vi "FPGA_Host_USB7855R.vi"() -> (8 "FilePath":path=path "D:/temp/test.tdms")   [LabVIEW 2023]
uses:
  <vilib>/rvi/interface/nirviReadWriteControl/nirviReadWriteControl.xnode
  <vilib>/rvi/interface/nirviMethod/nirviMethod.xnode
  User_Vi/Settings.vi
  <vilib>/rvi/interface/nirviOpenFPGA/nirviOpenFPGA.xnode
  <vilib>/rvi/errors/niLvFpgaMergeErrorWithErrorCode.vi
  <vilib>/rvi/errors/niLvFpgaAdjustHostInterfaceError.vi
  AllFiles_WEC-SPM-master/AllFiles_WEC-SPM-master/Sub_Vi/FPGA/FPGA_Target_USB_7855R.vi
  AllFiles_WEC-SPM-master/AllFiles_WEC-SPM-master/FPGA Bitfiles/wecspmusb7855r_FPGATargetUSB785_FPGATargetUSB785_scBLrgoL084.lvbitx
  <vilib>/FPGAPlugInAG/Dynamic/niLvFpga_Run_Dynamic.vi
  <vilib>/rvi/interface/Simulation/niFpgaSimulationCallBeginRW.vi
  <vilib>/FPGAPlugInAG/Dynamic/niLvFpga_WriteFifo_Dynamic.vi
  <vilib>/FPGAPlugInAG/Dynamic/niLvFpga_ReadFifo_Dynamic.vi
  <vilib>/FPGAPlugInAG/Dynamic/niLvFpga_StartFifo_Dynamic.vi
  <vilib>/FPGAPlugInAG/Dynamic/niLvFpga_StopFifo_Dynamic.vi
  TypeDefs/WayPointCluster.ctl
  TypeDefs/Settings.ctl
  TypeDefs/ChangeOnFly.ctl
  TypeDefs/Display.ctl
panel:
  in  "FPGA VI Reference Out":refnum<k20>
  out "error out 4":errorcluster
  out "error out 3":errorcluster
  out "Stop Hold Position":bool
  out "Applied Z":i16
  out "DIO0":bool
  out "error out 2":errorcluster
  out "error out":errorcluster
  out "ChangeonFlyUpdate":T1
  in  "Display Cluster":T2
  in  "ChangeonFly":T3
  in  "SettingsCluster":T4={"Sample Rate (us)"=1, "Samples Per Data Point (int, power of 2)"=1000, "DistanceToBulk (um)"=-1.0, "HoldTimeScaler"=1, "SaveData"=TRUE, "DistanceToBulk (um) 2"=-1.0, "DistanceToBulk (um) 3"=-1.0}
  in  "WayPointCluster":T5
  out "tdms file out":refnum<k34>
  out "ElementsToRead":u32=800
  in  "stop":bool
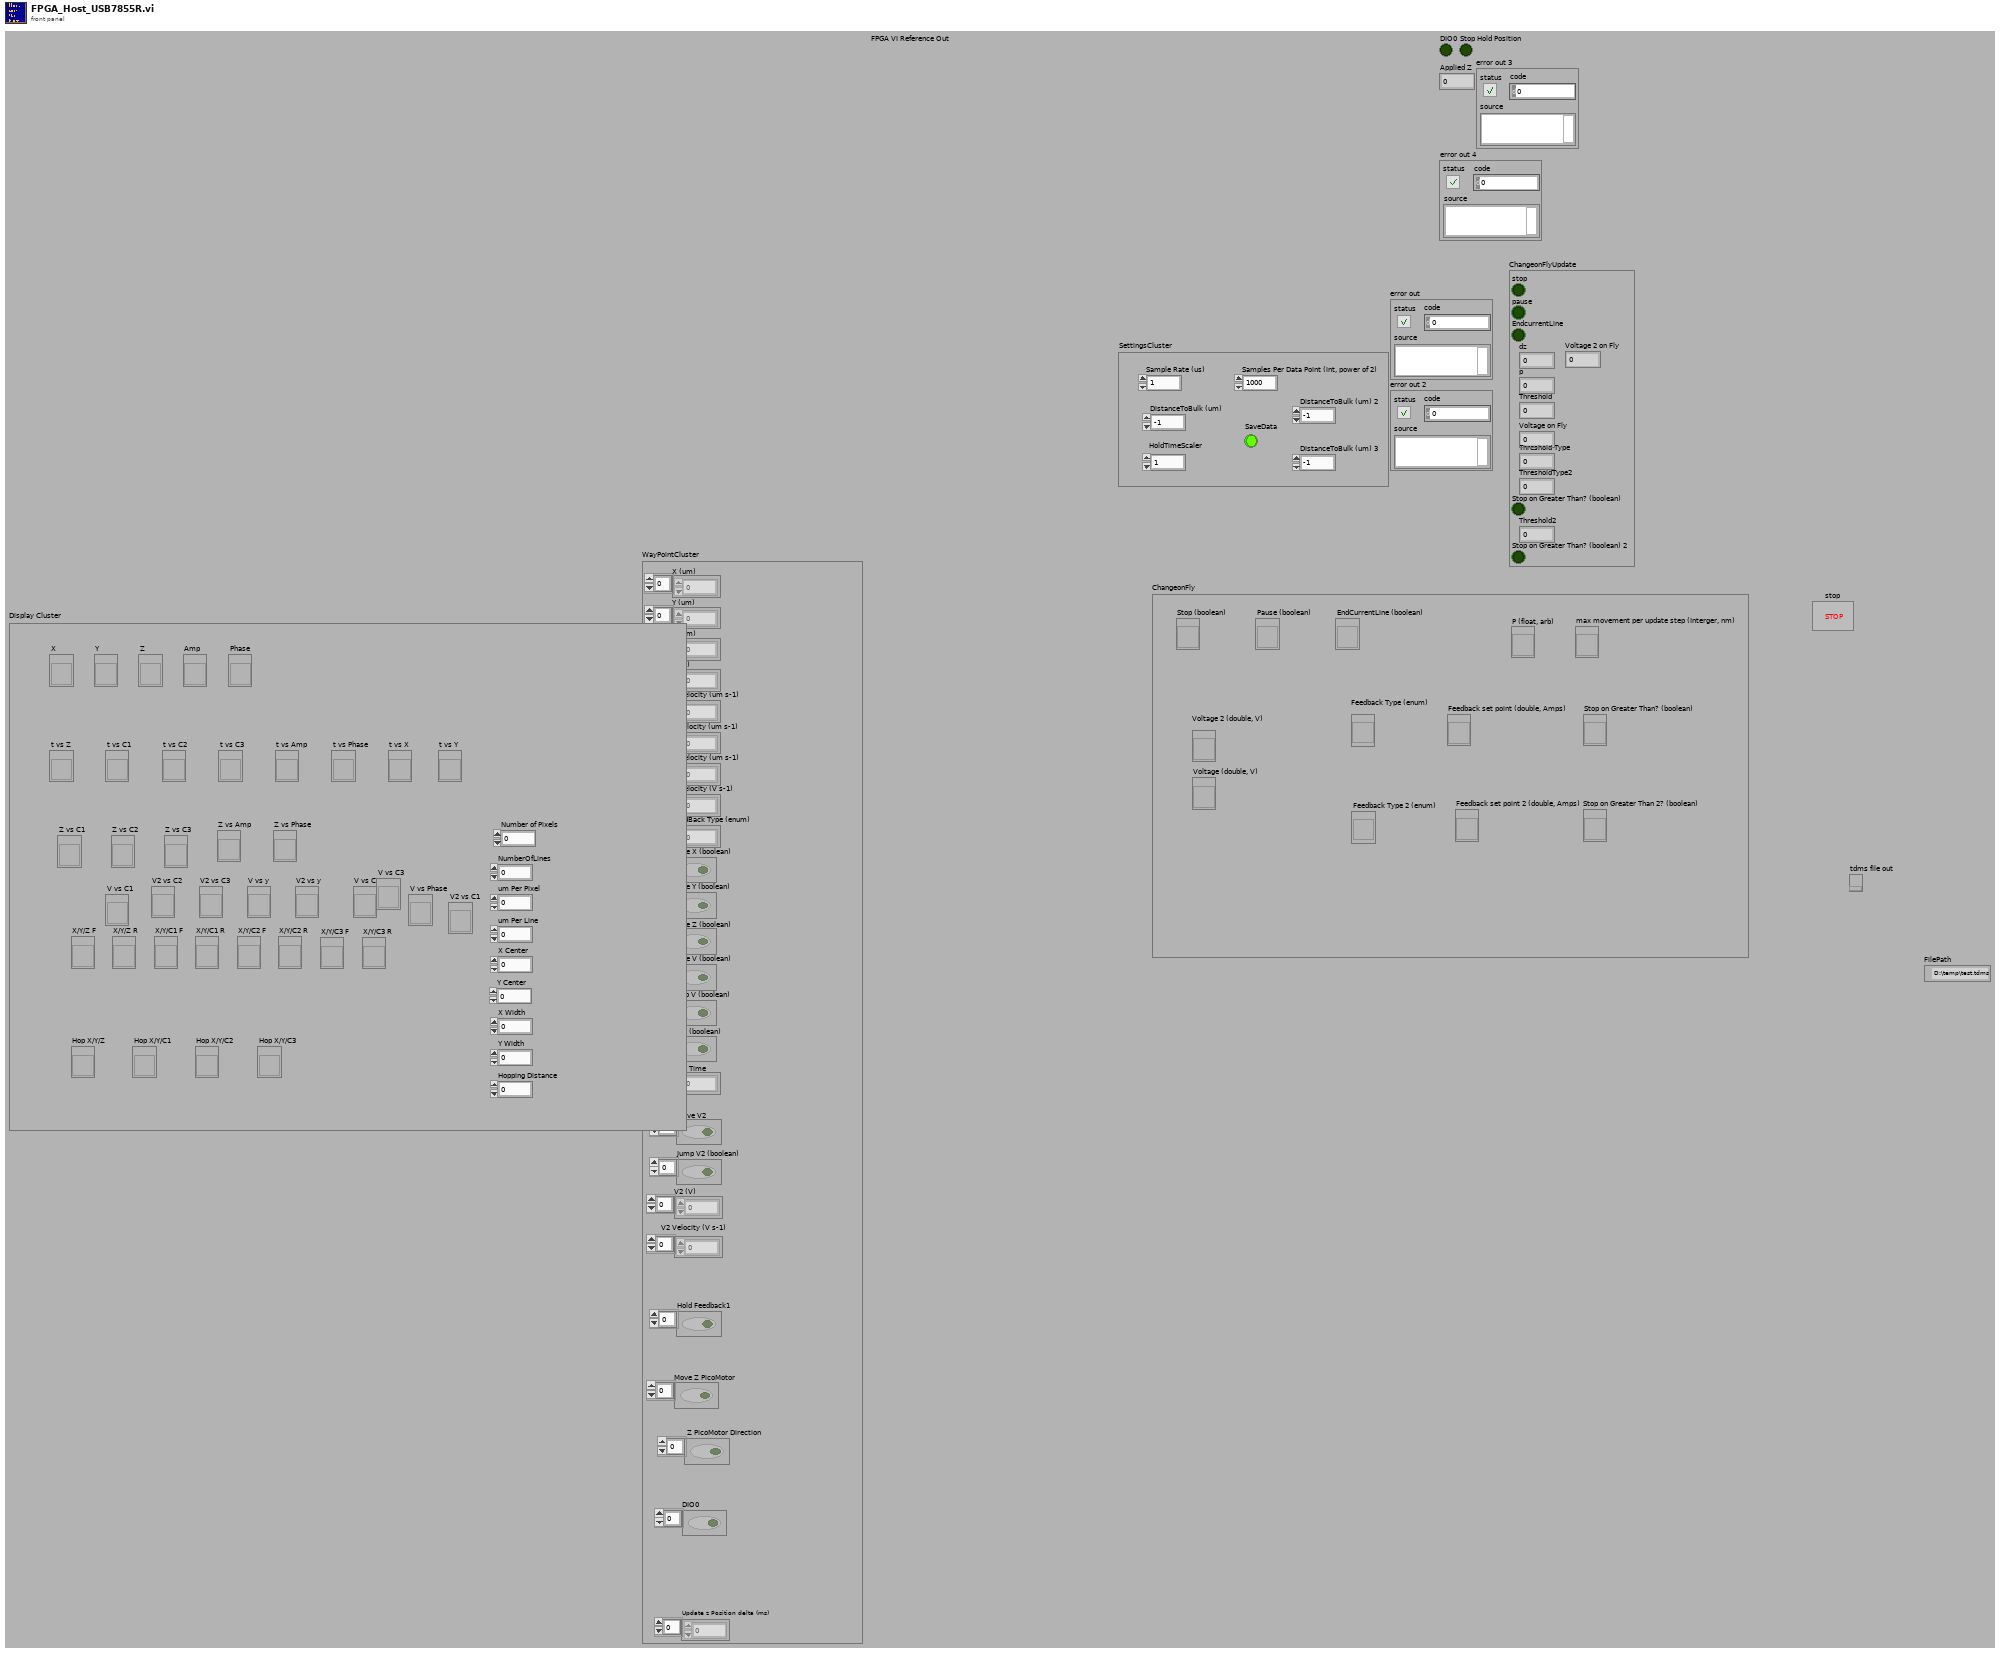
[diagram p1: front panel]
types:
  T1 = cluster{"stop":bool, "pause":bool, "EndcurrentLine":bool, "dz":i32, "p":fxp<+/-,32,1>, "Threshold":i32, "Voltage on Fly":i16, "Threshold Type":u8, "ThresholdType2":u8, "Stop on Greater Than? (boolean)":bool, "Threshold2":i32, "Stop on Greater Than? (boolean) 2":bool, "Voltage 2 on Fly":i16}
  T2 = typedef "Display.ctl" = cluster{"X":refnum<vi>, "Y":refnum<vi>, "Z":refnum<vi>, "Amp":refnum<vi>, "Phase":refnum<vi>, "t vs Z":refnum<vi>, "t vs C1":refnum<vi>, "t vs C2":refnum<vi>, "t vs C3":refnum<vi>, "t vs Amp":refnum<vi>, "t vs Phase":refnum<vi>, "t vs X":refnum<vi>, "t vs Y":refnum<vi>, "Z vs C1":refnum<vi>, "Z vs C2":refnum<vi>, "Z vs C3":refnum<vi>, "V vs C1":refnum<vi>, "V vs C2":refnum<vi>, "V vs C3":refnum<vi>, "X/Y/Z F":refnum<vi>, "X/Y/Z R":refnum<vi>, "X/Y/C1 F":refnum<vi>, "X/Y/C1 R":refnum<vi>, "X/Y/C2 F":refnum<vi>, "X/Y/C2 R":refnum<vi>, "X/Y/C3 F":refnum<vi>, "X/Y/C3 R":refnum<vi>, "NumberOfLines":u16, "um Per Pixel":dbl, "um Per Line":dbl, "X Center":dbl, "Hop X/Y/Z":refnum<vi>, "Hop X/Y/C1":refnum<vi>, "Hop X/Y/C2":refnum<vi>, "Hop X/Y/C3":refnum<vi>, "X Width":dbl, "Y Width":dbl, "Hopping Distance":dbl, "V2 vs C1":refnum<vi>, "V vs Phase":refnum<vi>, "Y Center":dbl, "Number of Pixels":dbl, "V2 vs C2":refnum<vi>, "V2 vs C3":refnum<vi>, "V vs y":refnum<vi>, "V2 vs y":refnum<vi>, "Z vs Amp":refnum<vi>, "Z vs Phase":refnum<vi>}
  T3 = typedef "ChangeOnFly.ctl" = cluster{"Stop (boolean)":refnum<vi>, "Pause (boolean)":refnum<vi>, "EndCurrentLine (boolean)":refnum<vi>, "max movement per update step (Interger, nm)":refnum<vi>, "P (float, arb)":refnum<vi>, "Feedback set point (double, Amps)":refnum<vi>, "Voltage (double, V)":refnum<vi>, "Feedback set point 2 (double, Amps)":refnum<vi>, "Stop on Greater Than 2? (boolean)":refnum<vi>, "Stop on Greater Than? (boolean)":refnum<vi>, "Voltage 2 (double, V)":refnum<vi>, "Feedback Type (enum)":refnum<vi>, "Feedback Type 2 (enum)":refnum<vi>}
  T4 = typedef "Settings.ctl" = cluster{"Sample Rate (us)":u32, "Samples Per Data Point (int, power of 2)":i16, "DistanceToBulk (um)":dbl, "HoldTimeScaler":u64, "SaveData":bool, "DistanceToBulk (um) 2":dbl, "DistanceToBulk (um) 3":dbl}
  T5 = typedef "WayPointCluster.ctl" = cluster{"X (um)":dbl[], "Y (um)":dbl[], "Z (um)":dbl[], "V (V)":dbl[], "X Velocity (um s-1)":dbl[], "Y Velocity (um s-1)":dbl[], "Z Velocity (um s-1)":dbl[], "V Velocity (V s-1)":dbl[], "FeedBack Type (enum)":u16[], "Move X (boolean)":bool[], "Move Y (boolean)":bool[], "Move Z (boolean)":bool[], "Move V (boolean)":bool[], "Jump V (boolean)":bool[], "Hold (boolean)":bool[], "Hold Time":u32[], "V2 (V)":dbl[], "Move V2":bool[], "V2 Velocity (V s-1)":dbl[], "Jump V2 (boolean)":bool[], "Update z Position delta (ms)":i16[], "Hold Feedback1":bool[], "Move Z PicoMotor":bool[], " Z PicoMotor Direction":bool[], "DIO0":bool[]}
  T6 = typedef "nirio_resource_hc.ctl" = tag
  T7 = typedef "VelScallerCluster.ctl" = cluster{"X_VelScaller":i32, "Y_VelScaller":i32, "Z_VelScaller":i32, "V s-1_VelScaller":i32, "V2 s-1_VelScaller":i32}
  T8 = enum16{"open", "open or create", "create or replace", "create", "open (read-only)"}
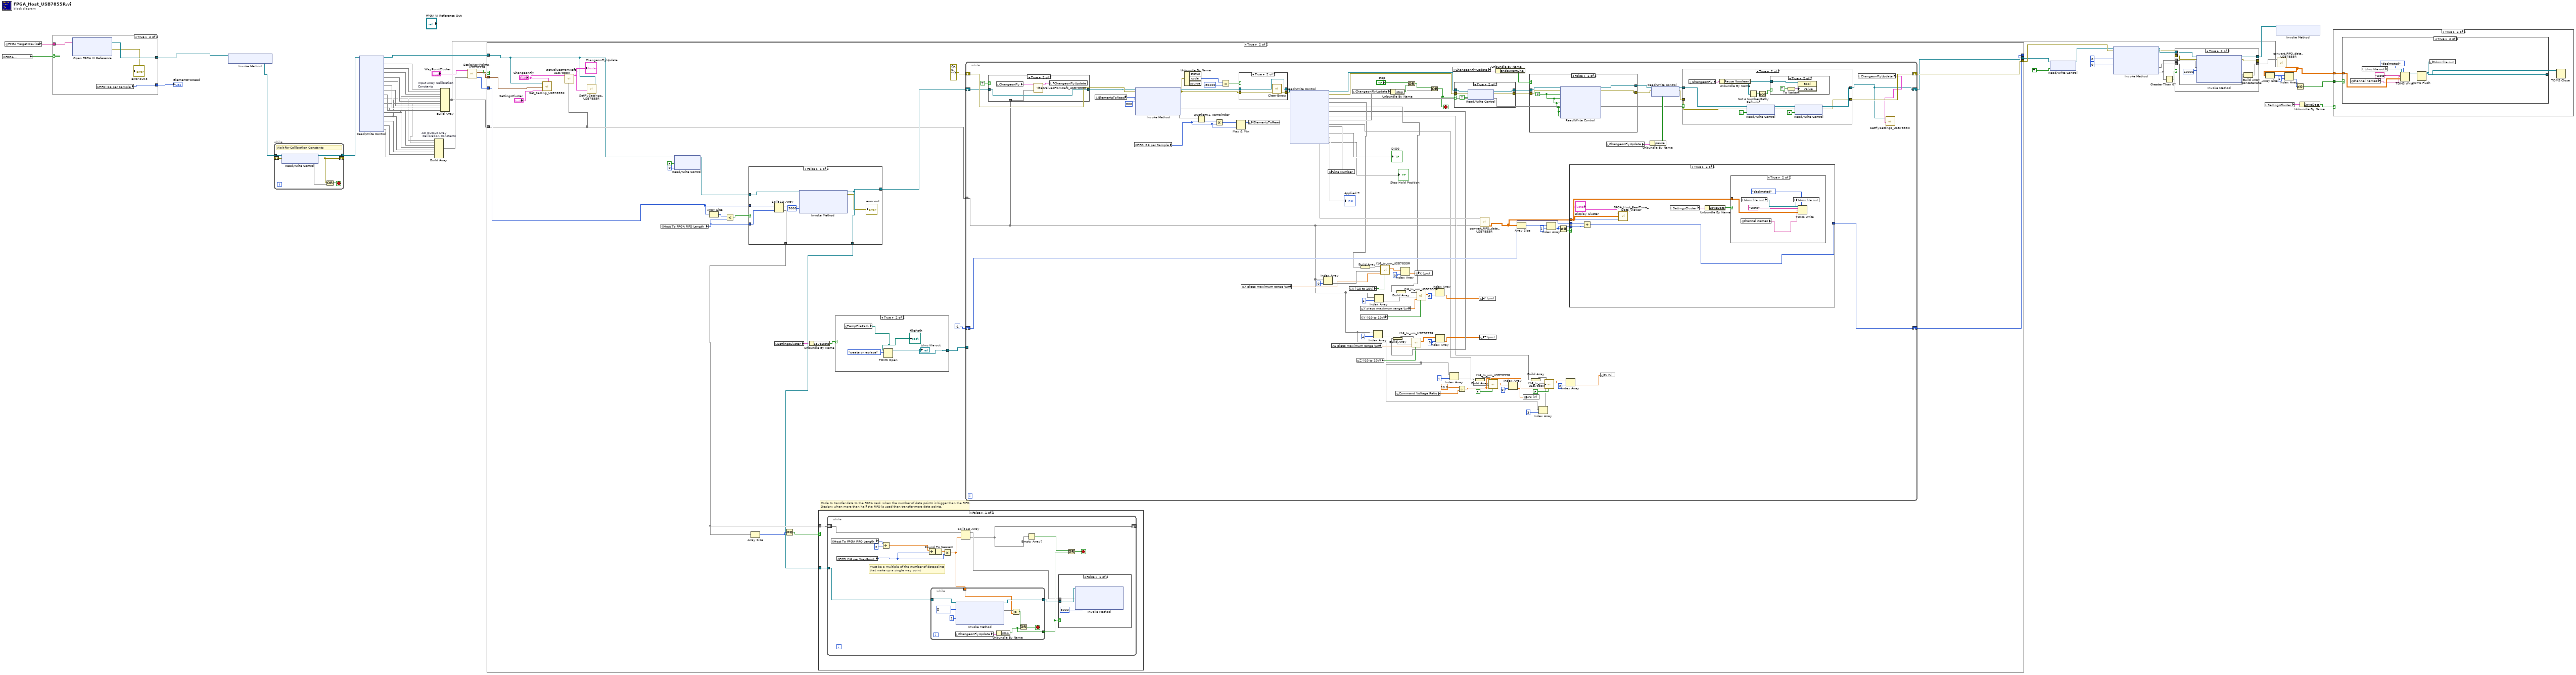
[diagram p0: block diagram]
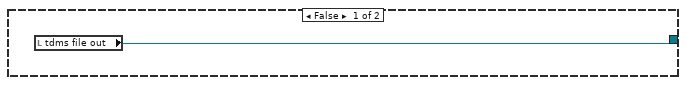
[diagram p3: hidden frame]
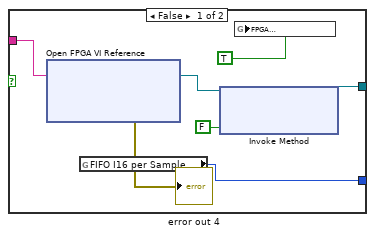
[diagram p4: hidden frame]
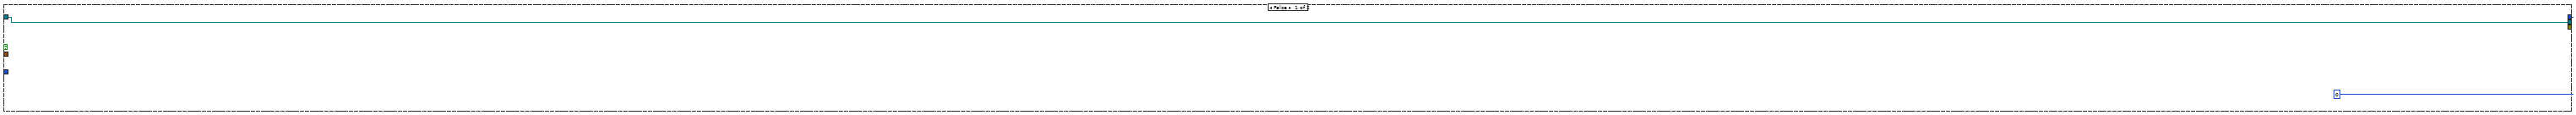
[diagram p6: hidden frame]
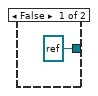
[diagram p7: hidden frame]
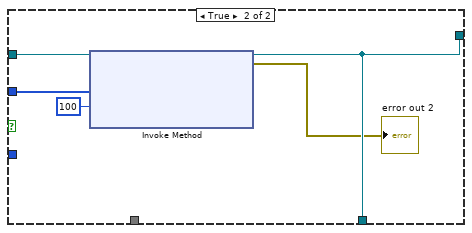
[diagram p10: hidden frame]
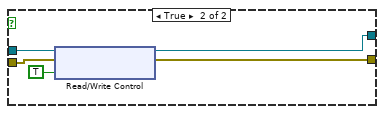
[diagram p14: hidden frame]
diagram:
  n1 = global read "Settings.vi" "FPGA \nrunning"() -> (w31:bool)
  n2 = global read "Settings.vi" "FPGA Target Device"() -> (w29:T6)
  n3 = case shown="True" w31 {
    tunnel: [w54 w60] -> w1
    tunnel: [w52 w59] -> w30
    tunnel: w29 -> [w51 w58]
    frame False {
      n4 = xnode "Open FPGA VI Reference"("resource name"=w51) -> ("FPGA VI Reference Out"=w55:refnum<k20>, "error out"=→"error out 4":errorcluster)  [unwired: 1 in]
      n5 = global read "Settings.vi" "FIFO I16 per Sample"() -> (w52:u32)
      n6 = xnode "Invoke Method"("FPGA VI Reference In"=w55, "Wait Until Done (F)"=FALSE) -> ("FPGA VI Reference Out"=w54:refnum<k20>)  [unwired: 1 in, 1 out]
      n7 = global write "Settings.vi" "FPGA \nrunning"(TRUE ("FPGA RUNNING")) -> ()
    }
    frame True {
      n8 = xnode "Open FPGA VI Reference"("resource name"=w58) -> ("FPGA VI Reference Out"=w60:refnum<k20>, "error out"=→"error out 3":errorcluster)  [unwired: 1 in]
      n9 = global read "Settings.vi" "FIFO I16 per Sample"() -> (w59:u32)
    }
  }
  "ElementsToRead" <- w30
  n10 = xnode "Invoke Method"("FPGA VI Reference In"=w1) -> ("FPGA VI Reference Out"=w3:refnum<k20>)  [unwired: 1 in, 1 out]
  n11 = while {
    tunnel: w3 -> [w66]
    tunnel: [w62] -> w2
    shift-right: [w61] -> _
    shift-left: _ -> [w65]
    stop <- w64 stop-if-true
    # "Wait for Calibration Constants"
    n12 = xnode "Read/Write Control"("FPGA VI Reference In"=w66, "error in"=w65) -> ("FPGA VI Reference Out"=w62:refnum<k20>, "error out"=w61:errorcluster, "CalConstants Ready"=w63)
    n13 = Compound Arithmetic op=OR(w61, w63) -> (w64:bool)
  }
  n14 = xnode "Read/Write Control"("FPGA VI Reference In"=w2) -> ("FPGA VI Reference Out"=w28:refnum<k20>, "CalCoefAi0"=w27, "CalCoefAi1"=w26, "CalCoefAi2"=w25, "CalCoefAi3"=w24, "CalCoefAi4"=w23, "CalCoefAi5"=w21, "CalCoefAi6"=w22, "CalCoefAi7"=w20, "CalCoefAo0"=w15, "CalCoefAo1"=w14, "CalCoefAo2"=w13, "CalCoefAo3"=w12, "CalCoefAo4"=w11, "CalCoefAo5"=w10, "CalCoefAo6"=w9, "CalCoefAo7"=w8)  [unwired: 1 in, 1 out]
  n15 = Build Array "AO Output Array\n Calibration Constants"(w15, w14, w13, w12, w11, w10, w9, w8) -> (w7:void[])
  n16 = Build Array "Input Array Calibration Constants"(w27, w26, w25, w12, w11, w24, w23, w22, w21, w20) -> (w4:void[])
  n17 = call "ScaleWayPoints_USB7855R.vi"("AO Calibration Constants"=w7, "WayPointCluster"="WayPointCluster") -> ("FPGA Way Points"=w17:i16[], "VelScallerCluster"=w16:T7, ".not. x?"=w18:bool)  [unwired: 7 in]
  n18 = case shown="True" w18 {
    tunnel: [w67 w78] -> w36
    tunnel: [_ w94] -> w49
    tunnel: w17 -> [_ w85]
    tunnel: [0 ("dimension size") w88] -> _
    tunnel: w28 -> [w67 w69]
    tunnel: w16 -> [_ w74]
    tunnel: w4 -> [_ w72]
    frame False {
    }
    frame True {
      # "Code to transfer data to the FPGA card, when the number of data points is bigger than the FIFO.\nDesign: when more than half the FIFO is used then transfer more data points."
      n19 = call "Set_Setting_USB7855R.vi"("ChangeonFly"="ChangeonFly", "SettingsCluster"="SettingsCluster", "VelScallerCluster"=w74, "FPGA VI Reference Out"=w69) -> ()  [unwired: 7 in, 1 out]
      n20 = call "GetValuesFromRefs_USB7855R.vi"("Array"=w72, "ChangeonFly"="ChangeonFly") -> ("output cluster"=w70:T1)  [unwired: 9 in]
      "ChangeonFlyUpdate" <- w70
      n21 = call "SetFlySettings_USB7855R.vi"("output cluster 3"=w70, "FPGA VI Reference Out"=w69) -> ()  [unwired: 10 in]
      n22 = global read "Settings.vi" "Host To FPGA FIFO Length"() -> (w75:i64)
      n23 = xnode "Read/Write Control"("FPGA VI Reference In"=w69, "External Stop"=FALSE, "LineNumber"=0) -> ("FPGA VI Reference Out"=w87:refnum<k20>)  [unwired: 1 in, 1 out]
      n24 = Array Size(array=w85) -> (size(s)=w84:i32)
      n25 = Less?(x=w84, y=w75) -> (x < y?=w83:bool)
      n26 = case shown="False" w83 {
        tunnel: w87 -> [w135 w141]
        tunnel: [w130 w138] -> w86
        tunnel: w85 -> [w134 w139]
        tunnel: w75 -> [w133 _]
        tunnel: [w131 _] -> w80
        tunnel: [w130 w138] -> w79
        frame False {
          n27 = Split 1D Array(array=w134, index=w133) -> (first subarray=w132:i16[], second subarray=w131:i16[])
          n28 = xnode "Invoke Method"("FPGA VI Reference In"=w135, "Data"=w132, "Timeout (ms)"=5000) -> ("FPGA VI Reference Out"=w130:refnum<k20>, "error out"=→"error out":errorcluster)  [unwired: 1 in, 1 out]
        }
        frame True {
          n29 = xnode "Invoke Method"("FPGA VI Reference In"=w141, "Data"=w139, "Timeout (ms)"=100) -> ("FPGA VI Reference Out"=w138:refnum<k20>, "error out"=→"error out 2":errorcluster)  [unwired: 1 in, 1 out]
        }
      }
      n30 = Array Size(array=w80) -> (size(s)=w82:i32)
      n31 = local read "SettingsCluster"() -> (w77:T4)
      n32 = Equal To 0?(x=w82) -> (x = 0?=w81:bool)
      n33 = Unbundle By Name(w77) -> ("SaveData"=w76:bool)
      n34 = case shown="False" w81 {
        tunnel: w80 -> [w100 _]
        tunnel: w79 -> [w99 _]
        frame False {
          n35 = while {
            shift-right: [w104] -> _
            shift-left: w100 -> [w115]
            tunnel: w99 -> [w107]
            stop <- w113 stop-if-true
            # "Must be a multiple of the number of datapoints \nthat make up a single way point"
            n36 = global read "Settings.vi" "Host To FPGA FIFO Length"() -> (w102:i64)
            n37 = global read "Settings.vi" "FIFO I16 per WayPoint"() -> (w101:i64)
            n38 = Divide(x=w102, y=i64 2) -> (x/y=w106:dbl)
            n39 = Divide(x=w106, y=w101) -> (x/y=w109:dbl)
            n40 = Round To Nearest(number=w109) -> (nearest integer value=w108:dbl)
            n41 = Multiply(x=w108, y=w101) -> (x*y=w105:dbl)
            n42 = while {
              tunnel: w107 -> [w122]
              tunnel: [w121] -> w112
              tunnel: [w125] -> w111
              tunnel: w105 -> [w119]
              stop <- w128 stop-if-true
              n43 = local read "ChangeonFlyUpdate"() -> (w126:T1)
              n44 = xnode "Invoke Method"("FPGA VI Reference In"=w122, "Data"=u64[] [], "Timeout (ms)"=1) -> ("FPGA VI Reference Out"=w121:refnum<k20>, "Empty Elements Remaining"=w120)  [unwired: 1 in, 1 out]
              n45 = Unbundle By Name(w126) -> ("stop"=w125:bool)
              n46 = Greater?(x=w120, y=w119) -> (0:w127:bool)
              n47 = Or(x=w127, y=w125) -> (x .or. y?=w128:bool)
            }
            n48 = Split 1D Array(array=w115, index=w105) -> (first subarray=w110:i16[], second subarray=w104:i16[])
            n49 = Empty Array?(array=w104) -> (empty?=w103:bool)
            n50 = case shown="False" w111 {
              tunnel: w112 -> [w117 _]
              tunnel: w110 -> [w116 _]
              frame False {
                n51 = xnode "Invoke Method"("FPGA VI Reference In"=w117, "Data"=w116, "Timeout (ms)"=5000) -> ()  [unwired: 1 in, 3 out]
              }
              frame True {
              }
            }
            n52 = Or(x=w103, y=w111) -> (x .or. y?=w113:bool)
          }
        }
        frame True {
        }
      }
      n53 = case shown="True" w76 {
        tunnel: [refnum<k34> refnum ("tdms file out") w98] -> w92
        frame False {
        }
        frame True {
          n54 = global read "Settings.vi" "TempFilePath"() -> (w96:path)
          "FilePath" <- w96
          n55 = TDMS Open(10:T8."create or replace" ("operation (0:open)"), 11:w96) -> (3:w98:refnum<k34>)  [unwired: 5 in, 1 out]
          "tdms file out" <- w98
        }
      }
      n56 = while {
        shift-right: [w203] -> w94
        shift-left: errorcluster {"status"=FALSE, "code"=0, "source"=""} ("error out") -> [w239]
        shift-right: [w145] -> w78
        shift-left: w86 -> [w207]
        shift-right: [w225] -> w88
        shift-left: -1 ("dimension size") -> [w235]
        tunnel: w92 -> [_]
        tunnel: w72 -> [w143]
        stop <- w199 stop-if-true
        n57 = case shown="True" TRUE {
          tunnel: w207 -> [w241 w245]
          tunnel: [w241 w245] -> w206
          tunnel: w143 -> [_ w242]
          frame False {
          }
          frame True {
            n58 = local read "ChangeonFly"() -> (w244:T3)
            n59 = call "GetValuesFromRefs_USB7855R.vi"("Array"=w242, "ChangeonFly"=w244) -> ("output cluster"=w243:T1)  [unwired: 9 in]
            n60 = local write "ChangeonFlyUpdate"(w243) -> ()
          }
        }
        n61 = local read "ElementsToRead"() -> (w227:u32)
        n62 = global read "Settings.vi" "FIFO I16 per Sample"() -> (w196:u32)
        n63 = xnode "Invoke Method"("FPGA VI Reference In"=w206, "error in"=w239, "Number of Elements"=w227, "Timeout (ms)"=800) -> ("FPGA VI Reference Out"=w229:refnum<k20>, "error out"=w228:errorcluster, "Data"=w195:void[], "Elements Remaining"=w226)
        n64 = Unbundle By Name(w228) -> ("code"=w238:i32)  [unwired: 2 out]
        n65 = Quotient & Remainder(x=w226, y=w196) -> (floor(x/y)=w222:u32)  [unwired: 1 out]
        n66 = Multiply(x=w222, y=w196) -> (x*y=w224:u32)
        n67 = Equal?(x=w238, y=-50400) -> (x = y?=w236:bool)
        n68 = Max & Min(x=w224, y=w196) -> (max(x,y)=w223:u32)  [unwired: 1 out]
        n69 = case shown="True" w236 {
          tunnel: w228 -> [w295 w298]
          tunnel: [w295 w297] -> w233
          tunnel: w229 -> [w294 w296]
          tunnel: [w294 w296] -> w232
          frame False {
          }
          frame True {
            n70 = call <vilib>:"Clear Errors.vi"("error in (no error)"=w298) -> ("error out"=w297:errorcluster)  [unwired: 5 in, 1 out]
          }
        }
        n71 = global read "Settings.vi" "X piezo maximum range (µm)"() -> (w189:dbl)
        n72 = local write "ElementsToRead"(w223) -> ()
        n73 = xnode "Read/Write Control"("FPGA VI Reference In"=w232, "error in"=w233) -> ("FPGA VI Reference Out"=w231:refnum<k20>, "error out"=w230:errorcluster, "Internal Pause"=w204, "CurrentMeasuredX"=w193, "CurrentMeasuredY"=w184, "CurrentMeasuredZ"=w174, "Applied Voltage"=w164, "WaitingForWayPoints"=w198, "Applied Voltage 2"=w163, "LineNumber"=w197, "DIO0"=→"DIO0", "Applied Z"=→"Applied Z", "Stop Hold Position"=→"Stop Hold Position")
        n74 = Index Array(array=w143, index=0) -> (element=w190)
        n75 = global write "Settings.vi" "Line Number"(w197) -> ()
        n76 = global read "Settings.vi" "Z piezo maximum range (µm)"() -> (w170:dbl)
        n77 = global read "Settings.vi" "X (-10 to 10V)"() -> (w188:bool)
        n78 = local read "ChangeonFlyUpdate"() -> (w202:T1)
        n79 = global read "Settings.vi" "Z (-10 to 10V)"() -> (w169:bool)
        n80 = global read "Settings.vi" "Y piezo maximum range (µm)"() -> (w179:dbl)
        n81 = global read "Settings.vi" "Y (-10 to 10V)"() -> (w178:bool)
        n82 = Build Array(w193) -> (w192:void[])
        n83 = Index Array(array=w143, index=2) -> (element=w167)
        n84 = Index Array(array=w143, index=1) -> (element=w176)
        n85 = call "I16_to_um_USB7855R.vi"("-10 to 10V range?"=w188, "Max Value [um]"=w189, "Channel Calibration"=w190, "Input_I16"=w192) -> ("output_um"=w187:dbl[])  [unwired: 7 in]
        n86 = Unbundle By Name(w202) -> ("stop"=w214:bool)
        n87 = Build Array(w174) -> (w173:void[])
        n88 = global read "Settings.vi" "Command Voltage Ratio"() -> (w154:dbl)
        n89 = Build Array(w184) -> (w183:void[])
        n90 = Index Array(array=w187, index=0) -> (element=w185:dbl)
        n91 = Or(x="stop", y=w214) -> (x .or. y?=w213:bool)
        n92 = call "I16_to_um_USB7855R.vi"("-10 to 10V range?"=w169, "Max Value [um]"=w170, "Channel Calibration"=w167, "Input_I16"=w173) -> ("output_um"=w172:dbl[])  [unwired: 7 in]
        n93 = global write "Settings.vi" "X (µm)"(w185) -> ()
        n94 = call "I16_to_um_USB7855R.vi"("-10 to 10V range?"=w178, "Max Value [um]"=w179, "Channel Calibration"=w176, "Input_I16"=w183) -> ("output_um"=w181:dbl[])  [unwired: 7 in]
        n95 = Or(x=w213, y=w198) -> (x .or. y?=w199:bool)
        n96 = Index Array(array=w181, index=0) -> (element=w180:dbl)
        n97 = Index Array(array=w172, index=0) -> (element=w171:dbl)
        n98 = Index Array(array=w143, index=4) -> (element=w150)
        n99 = local read "ChangeonFlyUpdate"() -> (w201:T1)
        n100 = case shown="True" w199 {
          tunnel: [w287 w293] -> w217
          tunnel: [w288 w292] -> w215
          tunnel: w230 -> [w288 w291]
          tunnel: w231 -> [w287 w289]
          frame False {
          }
          frame True {
            n101 = xnode "Read/Write Control"("FPGA VI Reference In"=w289, "error in"=w291, "External Stop"=TRUE ("Stop")) -> ("FPGA VI Reference Out"=w293:refnum<k20>, "error out"=w292:errorcluster)
          }
        }
        n102 = Divide(x=10.0 ("Max Value [um]"), y=w154) -> (x/y=w152:dbl)
        n103 = Build Array(w163) -> (w166:void[])
        n104 = global write "Settings.vi" "Y (µm)"(w180) -> ()
        n105 = global write "Settings.vi" "Z (µm)"(w171) -> ()
        n106 = call "convert_FIFO_data_USB7855R.vi"("Actual Data"=w195, "Calinbration Costants"=w143) -> ("appended array"=w194:dbl[][])  [unwired: 17 in]
        n107 = call "I16_to_um_USB7855R.vi"("-10 to 10V range?"=FALSE, "Max Value [um]"=w152, "Channel Calibration"=w150, "Input_I16"=w166) -> ("output_um"=w160:dbl[])  [unwired: 7 in]
        n108 = Unbundle By Name(w201) -> ("EndcurrentLine"=w212:bool)
        n109 = Index Array(array=w160, index=0) -> (element=w157:dbl)
        n110 = Array Size(array=w194) -> (size(s)=w221:i32[])
        n111 = global write "Settings.vi" "V2 (V)"(w157) -> ()
        n112 = case shown="False" w212 {
          tunnel: w217 -> [w267 w272]
          tunnel: [w266 w271] -> w216
          tunnel: w215 -> [w265 w270]
          tunnel: [w264 w269] -> w209
          frame False {
            w263 = FALSE ("OnlyStopLineONCE")
            n113 = xnode "Read/Write Control"("FPGA VI Reference In"=w267, "error in"=w265, "OnlyStopLineONCE V"=w263, "OnlyStopLineONCE Z"=w263, "OnlyStopLineONCE Y"=w263, "OnlyStopLineONCE X"=w263, "EndCurrentLine"=w263, "OnlyStopLineONCE V2"=w263) -> ("FPGA VI Reference Out"=w266:refnum<k20>, "error out"=w264:errorcluster)
          }
          frame True {
            n114 = xnode "Read/Write Control"("FPGA VI Reference In"=w272, "error in"=w270, "EndCurrentLine"=TRUE) -> ("FPGA VI Reference Out"=w271:refnum<k20>, "error out"=w269:errorcluster)
          }
        }
        n115 = Build Array(w164) -> (w165:void[])
        n116 = Index Array(array=w143, index=3) -> (element=w148)
        n117 = call "I16_to_um_USB7855R.vi"("-10 to 10V range?"=FALSE, "Max Value [um]"=w152, "Channel Calibration"=w148, "Input_I16"=w165) -> ("output_um"=w159:dbl[])  [unwired: 7 in]
        n118 = Index Array(array=w221, index=1) -> (element=w218:i32)
        n119 = Not Equal To 0?(x=w218) -> (x != 0?=w219:bool)
        n120 = Index Array(array=w159, index=0) -> (element=w158:dbl)
        n121 = case shown="True" w219 {
          tunnel: w235 -> [w273 w279]
          tunnel: [w273 w278] -> w225
          tunnel: w194 -> [_ w276]
          tunnel: w218 -> [_ w280]
          frame False {
          }
          frame True {
            n122 = Add(x=w279, y=w280) -> (x+y=w278:i32)
            n123 = call "FPGA_Host_RealTime_Data_Viewer.vi"("length"=w279, "Array"=w276, "Display Cluster"="Display Cluster") -> ()  [unwired: 3 in]
            n124 = local read "SettingsCluster"() -> (w275:T4)
            n125 = Unbundle By Name(w275) -> ("SaveData"=w274:bool)
            n126 = case shown="True" w274 {
              tunnel: w276 -> [_ w286]
              frame False {
              }
              frame True {
                n127 = global read "Settings.vi" "channel names"() -> (w281:string[])
                n128 = local read "tdms file out"() -> (w285:refnum<k34>)
                n129 = TDMS Write(0:w285, 1:enum16{"decimated", "interleaved"}."decimated" ("data layout (0:decimated)"), 5:"Data" ("group name in (Untitled)"), 7:w281, 9:w286) -> (4:w284:refnum<k34>)  [unwired: 1 in, 3 out]
                n130 = local write "tdms file out"(w284) -> ()
              }
            }
          }
        }
        n131 = global write "Settings.vi" "V (V)"(w158) -> ()
        n132 = local read "ChangeonFlyUpdate"() -> (w200:T1)
        n133 = Unbundle By Name(w200) -> ("pause"=w210:bool)
        n134 = xnode "Read/Write Control"("FPGA VI Reference In"=w216, "error in"=w209, "External Pause"=w210) -> ("FPGA VI Reference Out"=w211:refnum<k20>, "error out"=w208:errorcluster)
        n135 = case shown="True" w204 {
          tunnel: w211 -> [w247 w259]
          tunnel: [w247 w256] -> w145
          tunnel: w208 -> [w246 w254]
          tunnel: [w246 w252] -> w203
          frame False {
          }
          frame True {
            n136 = local read "ChangeonFly"() -> (w248:T3)
            n137 = Unbundle By Name(w248) -> ("Pause (boolean)"=w250:refnum<vi>)
            n138 = xnode "Read/Write Control"("FPGA VI Reference In"=w259, "error in"=w254, "External Pause"=TRUE) -> ("FPGA VI Reference Out"=w257:refnum<k20>, "error out"=w253:errorcluster)
            n139 = Not A Number/Path/Refnum?(number/path/refnum=w250) -> (NaN/Path/Refnum?=w251:bool)
            n140 = Not(x=w251) -> (.not. x?=w249:bool)
            n141 = case shown="True" w249 {
              tunnel: w250 -> [_ w260]
              frame False {
              }
              frame True {
                n142 = To Variant(anything=TRUE) -> (Variant=w261:variant)
                n143 = property on="Property Node" class="Bool"(reference=w260, "Value"=w261) -> ()  [unwired: 1 in, 2 out]
              }
            }
            n144 = xnode "Read/Write Control"("FPGA VI Reference In"=w257, "error in"=w253, "Internal Pause"=FALSE) -> ("FPGA VI Reference Out"=w256:refnum<k20>, "error out"=w252:errorcluster)
          }
        }
        n145 = local read "ChangeonFlyUpdate"() -> (w146:T1)
        n146 = call "SetFlySettings_USB7855R.vi"("output cluster 3"=w146, "FPGA VI Reference Out"=w145) -> ()  [unwired: 10 in]
      }
    }
  }
  n147 = xnode "Read/Write Control"("FPGA VI Reference In"=w36, "External Stop"=TRUE) -> ("FPGA VI Reference Out"=w34:refnum<k20>)  [unwired: 1 in, 1 out]
  n148 = xnode "Invoke Method"("FPGA VI Reference In"=w34, "error in"=w49, "Number of Elements"=u32 0, "Timeout (ms)"=0) -> ("FPGA VI Reference Out"=w43:refnum<k20>, "error out"=w38:errorcluster, "Data"=w44:void[], "Elements Remaining"=w45)
  n149 = Greater Than 0?(x=w45) -> (x > 0?=w46:bool)
  n150 = case shown="True" w46 {
    tunnel: w43 -> [w299 w310]
    tunnel: w45 -> [_ w309]
    tunnel: w44 -> [w301 w307]
    tunnel: [w301 w305] -> w6
    tunnel: w38 -> [w300 w304]
    tunnel: [w300 w303] -> _
    tunnel: [w299 w302] -> w37
    frame False {
    }
    frame True {
      n151 = xnode "Invoke Method"("FPGA VI Reference In"=w310, "error in"=w304, "Number of Elements"=w309, "Timeout (ms)"=10000) -> ("FPGA VI Reference Out"=w302:refnum<k20>, "error out"=w303:errorcluster, "Data"=w306:void[])  [unwired: 1 out]
      n152 = Build Array (concatenate)(w307, w306) -> (w305:void[])
    }
  }
  n153 = local read "SettingsCluster"() -> (w33:T4)
  n154 = xnode "Invoke Method"("FPGA VI Reference In"=w37) -> ()  [unwired: 1 in, 2 out]
  n155 = call "convert_FIFO_data_USB7855R.vi"("Actual Data"=w6, "Calinbration Costants"=w4) -> ("appended array"=w5:dbl[][])  [unwired: 17 in]
  n156 = Array Size(array=w5) -> (size(s)=w42:i32[])
  n157 = Index Array(array=w42, index=1) -> (element=w40:i32)
  n158 = Not Equal To 0?(x=w40) -> (x != 0?=w39:bool)
  n159 = Unbundle By Name(w33) -> ("SaveData"=w32:bool)
  n160 = case shown="True" w32 {
    tunnel: w39 -> [_ w313]
    tunnel: w5 -> [_ w312]
    frame False {
    }
    frame True {
      n161 = case shown="True" w313 {
        tunnel: w312 -> [_ w321]
        tunnel: [w314 w316] -> w311
        frame False {
          n162 = local read "tdms file out"() -> (w314:refnum<k34>)
        }
        frame True {
          n163 = global read "Settings.vi" "channel names"() -> (w315:string[])
          n164 = local read "tdms file out"() -> (w319:refnum<k34>)
          n165 = TDMS Write(0:w319, 1:enum16{"decimated", "interleaved"}."decimated" ("data layout (0:decimated)"), 5:"Data" ("group name in (Untitled)"), 7:w315, 9:w321) -> (4:w318:refnum<k34>)  [unwired: 1 in, 3 out]
          n166 = TDMS Flush(7:w318) -> (3:w316:refnum<k34>)  [unwired: 1 in, 1 out]
          n167 = local write "tdms file out"(w316) -> ()
        }
      }
      n168 = TDMS Close(11:w311) -> ()  [unwired: 1 in, 2 out]
    }
  }
